vi "main_ctrl.vi"(8 "error in":errorcluster) -> (0 "error out":errorcluster caption="Error")   [LabVIEW 2013]
uses:
  <vilib>/Rock Robotics/WPI/DriverStation/WPI_DriverStationRobotMode2.ctl
  typedefs/Test/test data.ctl
  typedefs/Test/test controls.ctl
  typedefs/fg_typedef.ctl
  typedefs/Vision/vision enable.ctl
  typedefs/State Machine/subStates.ctl
  typedefs/State Machine/singleUseSubstate.ctl
  <vilib>/Rock Robotics/WPI/Solenoid/WPI_SolenoidValue.ctl
  <vilib>/Rock Robotics/WPI/Compressor/WPI_CompressorGetSetRefNum.vi
  <vilib>/Rock Robotics/WPI/RobotDrive/WPI_RobotDriveGetSetRefNum.vi
  <vilib>/Rock Robotics/WPI/RobotDrive/WPI_RobotDriveArcadeDrive_Standard(NoSaturation).vi
  <vilib>/Rock Robotics/WPI/Solenoid/WPI_SolenoidSetEnum.vi
  state machine master/Cancel State Machine - Pickup.vi
  state machine master/Cancel State Machine - Load.vi
  typedefs/Vision/vision data.ctl
panel:
  in  "Test\nControls":T1 {"Belts" scale=-1.0..1.0; "Arm" scale=-1.0..1.0; "Drive Train" scale=-1.0..1.0}
  out "Test Data":T2
  out "Robot Mode":T3
  out "Vision SPI":u32
  out "Vision IPS":dbl
  out "Main IPS":dbl
  out "Main SPI":u32
  # "Test Input/Output"
  # "MAIN CONTROL"
  # "holds robot control code - dual parallel state machine"
  # "SPI: milliseconds per iteration\nIPS: iterations per second"
  # "Pneumatics"
  # "Home Encoders"
  # "Manual Override"
  # "Joystick Control"
  # "Arm Safeties"
  # "Sensors"
  # "Drive Encoders"
  # "Pneumatics Commands"
  # "Arm Encoder"
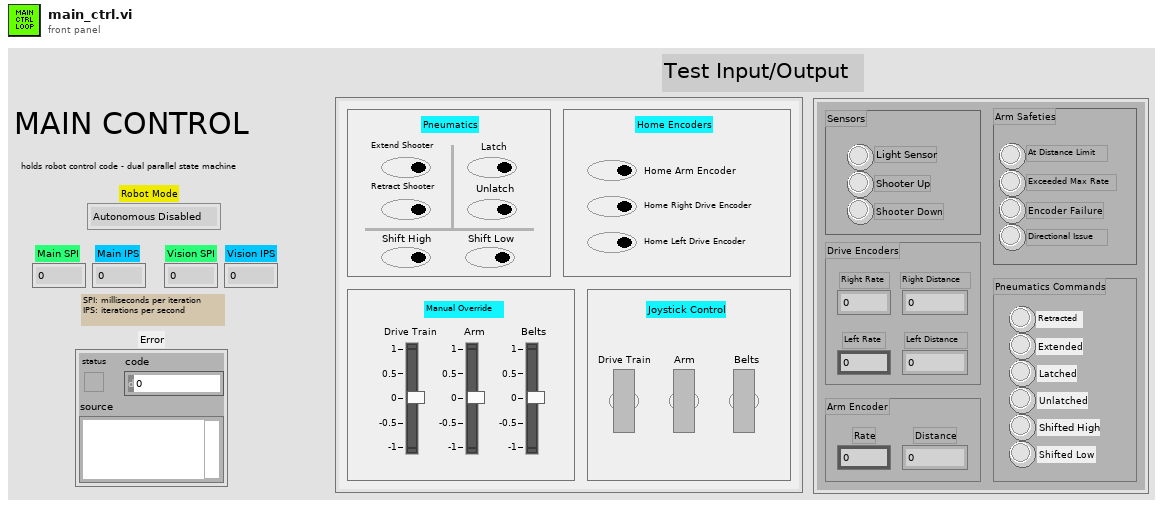
[diagram p1: front panel]
types:
  T1 = typedef "test controls.ctl" = cluster{"Drive Train":dbl, "Arm":dbl, "Belts":dbl, "Drive Train":bool, "Arm":bool, "Belts":bool, "Home Arm Encoder":bool, "Home Right Drive Encoder":bool, "Home Left Drive Encoder":bool, "Extend Shooter":bool, "Retract Shooter":bool, "Latch":bool, "Unlatch":bool, "Shift High":bool, "Shift Low":bool}
  T2 = typedef "test data.ctl" = cluster{"Light Sensor":bool, "Shooter Up":bool, "Shooter Down":bool, "Left Rate":dbl, "Left Distance":dbl, "Right Rate":dbl, "Right Distance":dbl, "Rate":dbl, "Distance":dbl, "At Distance Limit":bool, "Exceeded Max Rate":bool, "Encoder Failure":bool, "Directional Issue":bool, "Latched":bool, "Unlatched":bool, "Shifted High":bool, "Shifted Low":bool, "Extended":bool, "Retracted":bool}
  T3 = typedef "WPI_DriverStationRobotMode2.ctl" = enum16{"Autonomous Disabled", "Autonomous Enabled", "Teleop Disabled", "Teleop Enabled", "Timeout", "Finish", "Test Disabled", "Test Enabled"}
  T4 = typedef "fg_typedef.ctl" = enum16{"Get", "Set"}
  T5 = typedef "vision data.ctl" = cluster{"x":dbl, "y":dbl, "area":dbl, "width":dbl, "height":dbl, "Hot Goal Present?":bool, "distance":dbl}
  T6 = typedef "vision enable.ctl" = enum16{"Enable", "Disable", "Stop"}
  T7 = typedef "WPI_CameraDevRef.ctl" = cluster{"Camera Address":string, "CameraStatus":errorcluster, "Acquire Image Notifier":refnum<notifier>}
  T8 = typedef "IMAQ Image.ctl" = refnum<image>
  T9 = cluster{"Vision mSPI":u32, "Main mSPI":u32, "Dash mSPI":u32}
  T10 = typedef "WPI_RobotDriveDevRef.ctl" = cluster{"DevStatus":errorcluster, "Motors[]":T11[], "Square Inputs":bool, "Max Output":dbl, "Isochronous":bool}
  T11 = typedef "WPI_MotorControlDeviceRef.ctl" = cluster{"DeviceStatus":errorcluster, "Type":enum16{"PWM", "CAN"}, "PWM":cluster{"Digital Module":T12, "PWM Channel":T13, "DeadBand":T14}, "CAN":cluster{"Device Number":u8, "Control Mode":T15, "Semaphore":T16, "Max Vout":dbl}, "Invert":bool, "TransformRef":T17, "InvTransformRef":T17}
  T12 = typedef "FPGA_TypedefDigitalModule.ctl" = enum16{"Digital Module 1", "Digital Module 2"}
  T13 = typedef "FPGA_DIOPWMChannel.ctl" = enum8{"PWM 1", "PWM 2", "PWM 3", "PWM 4", "PWM 5", "PWM 6", "PWM 7", "PWM 8", "PWM 9", "PWM 10", "Invalid"}
  T14 = typedef "WPI_PWMDeadband.ctl" = cluster{"Name":string, "maxPositivePwm":i32, "minPositivePwm":i32, "centerPwm":i32, "maxNegativePwm":i32, "minNegativePwm":i32, "angularRange":u16}
  T15 = typedef "WPI_CANJaguar_ControlMode.ctl" = enum8{"Percent VBus", "Current", "Speed", "Position", "Voltage"}
  T16 = typedef "Semaphore RefNum" = refnum<k1>
  T17 = typedef "WPI_PWMTransform_ConPane.ctl" = refnum<vi>
  T18 = typedef "WPI_SolenoidDevRef.ctl" = cluster{"DevStatus":errorcluster, "Solenoid Module":T19, "Forward Solenoid Channel":T20, "Reverse Solenoid Channel":T20}
  T19 = typedef "FPGA_TypedefSolenoidModule.ctl" = enum16{"Solenoid Module 1", "Solenoid Module 2"}
  T20 = typedef "WPI_SolenoidChannel.ctl" = enum8{"Solenoid 1", "Solenoid 2", "Solenoid 3", "Solenoid 4", "Solenoid 5", "Solenoid 6", "Solenoid 7", "Solenoid 8", "Invalid"}
  T21 = typedef "WPI_CompressorDevRef.ctl" = cluster{"DevStatus":errorcluster, "DigitalInputDevRef":T22, "RelayDevRef":T24}
  T22 = typedef "WPI_DigitalInputDevRef.ctl" = cluster{"DevStatus":errorcluster, "DIO Channel":T23, "Digital Module":T12}
  T23 = typedef "FPGA_DIOChannel.ctl" = enum8{"DIO 1", "DIO 2", "DIO 3", "DIO 4", "DIO 5", "DIO 6", "DIO 7", "DIO 8", "DIO 9", "DIO 10", "DIO 11", "DIO 12", "DIO 13", "DIO 14", "Invalid"}
  T24 = typedef "WPI_RelayDevRef.ctl" = cluster{"DevStatus":errorcluster, "Relay Channel":T25, "Digital Module":T12, "Relay Direction":T26}
  T25 = typedef "FPGA_DIORelayChannel.ctl" = enum8{"Relay 1", "Relay 2", "Relay 3", "Relay 4", "Relay 5", "Relay 6", "Relay 7", "Relay 8", "Invalid"}
  T26 = typedef "WPI_RelayDirection.ctl" = enum16{"Both directions", "Forward only", "Reverse only"}
  T27 = typedef "WPI_SolenoidValue.ctl" = enum16{"Off", "On", "Forward", "Reverse"}
  T28 = typedef "singleUseSubstate.ctl" = enum16{"null", "wait", "shift high", "shift low", "extend shooter", "retract shooter", "latch", "unlatch", "end"}
  T29 = typedef "WPI_DriverStationDerivedRobotMode.ctl" = enum16{"Init", "Execute", "Stop"}
  T30 = typedef "subStates.ctl" = enum16{"null", "wait", "driver control", "auto", "manual override", "hold position", "rotate", "pickup", "pass", "load", "goto shoot", "shoot high goal", "shoot low goal", "cancel arm", "cancel shooter", "end", "test"}
  T31 = typedef "Loop 2 Datatype.ctl" = cluster{"State":T30, "Waiting Loop":i32, "State to Wait For":i32, "Loop ID":i32, "Exit Value":i32, "Joystick Y":dbl, "Joystick Z":dbl}
  T32 = typedef "Loop 1 Datatype.ctl" = cluster{"State":T30, "Waiting Loop":i32, "State to Wait For":i32, "Loop ID":i32, "Exit Value":i32}
  T33 = typedef "Loop 3 Datatype.ctl" = cluster{"State":T30, "Waiting Loop":i32, "State to Wait For":i32, "Loop ID":i32, "Exit Value":i32, "Joystick Y":dbl, "Tune Setpoint":cluster{"Increment":bool, "Decrement":bool}}
  T34 = typedef "Loop 0 Datatype.ctl" = cluster{"State":T30, "Waiting Loop":i32, "State to Wait For":i32, "Loop ID":i32, "Exit Value":i32, "X Axis":dbl, "Y Axis":dbl, "Z Axis":dbl}
  T35 = typedef "dashboard safety status data.ctl" = cluster{"At Distance Limit":bool, "Encoder Error":bool, "Excedded Rate Limit":bool, "Encoder Directional Issue":bool}
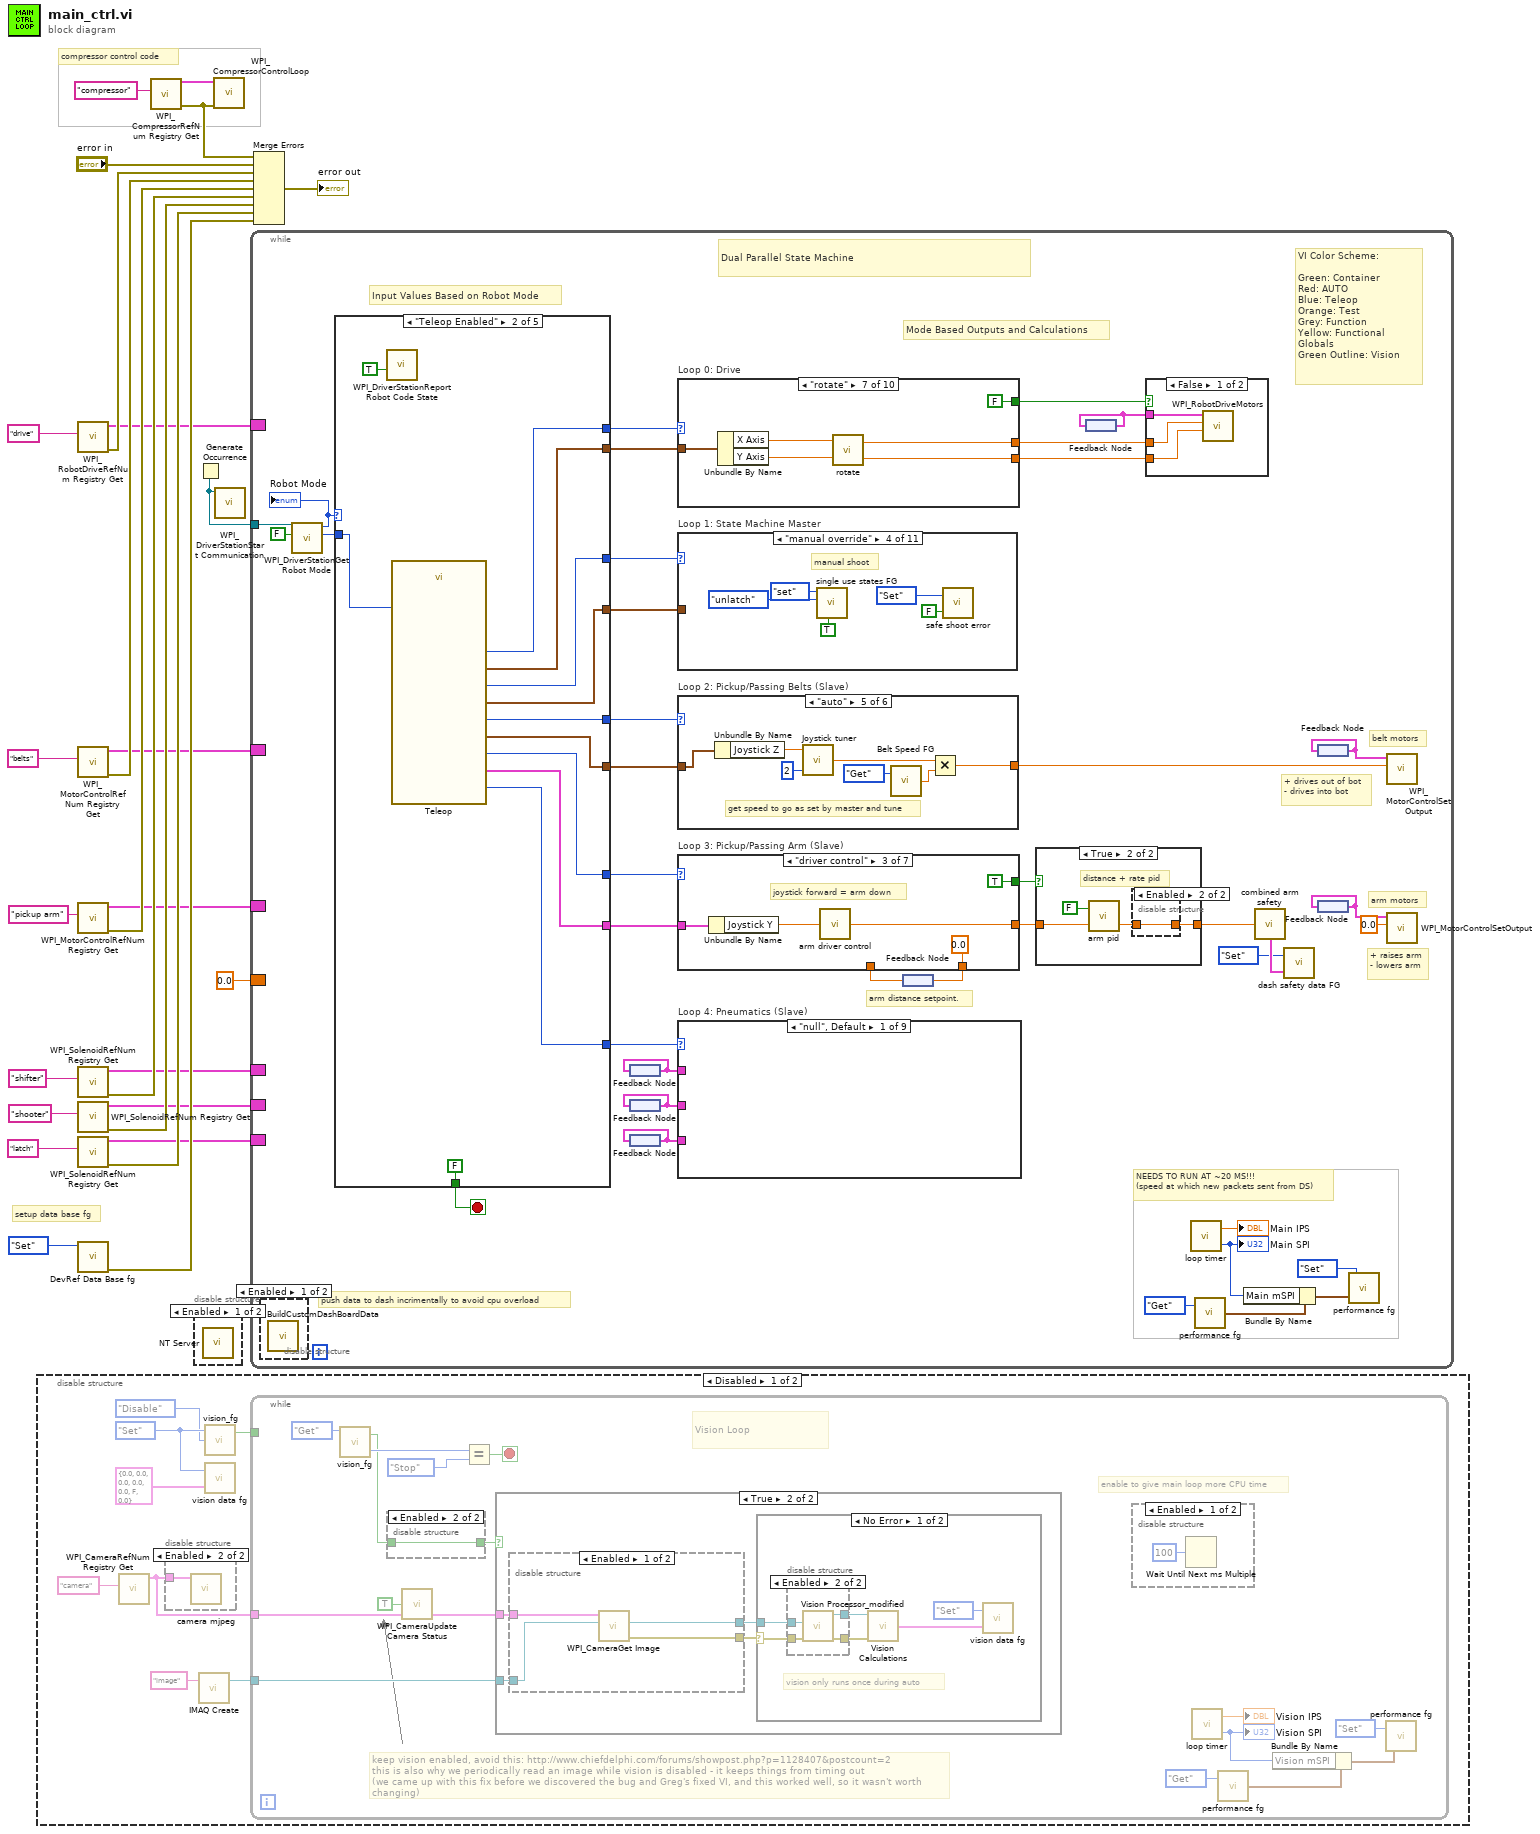
[diagram p0: block diagram]
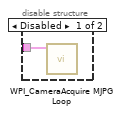
[diagram p3: hidden frame]
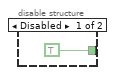
[diagram p4: hidden frame]
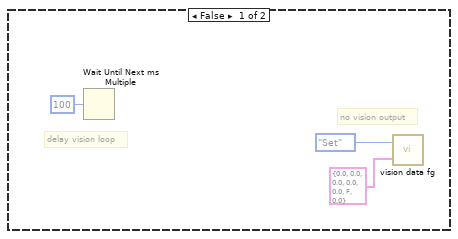
[diagram p6: hidden frame]
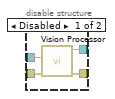
[diagram p7: hidden frame]
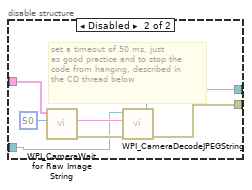
[diagram p9: hidden frame]
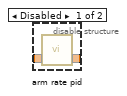
[diagram p12: hidden frame]
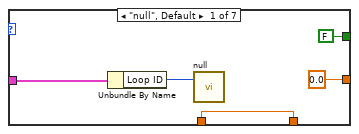
[diagram p13: hidden frame]
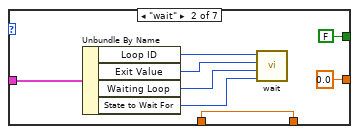
[diagram p14: hidden frame]
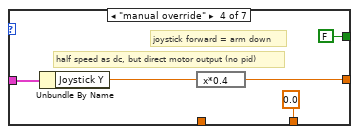
[diagram p15: hidden frame]
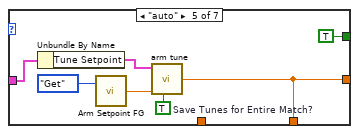
[diagram p16: hidden frame]
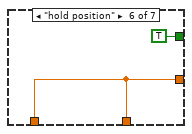
[diagram p17: hidden frame]
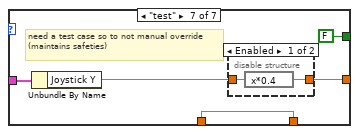
[diagram p18: hidden frame]
diagram:
  # "compressor control code"
  # "setup data base fg"
  n1 = disable-structure shown="Disabled" {
    frame Disabled {
      w33 = fg_typedef."Set" ("Enum")
      n2 = call <vilib>:"WPI_CameraRefNum Registry Get.vi"("refnum name"="camera") -> ("CameraDevRef"=w30:T7)  [unwired: 9 in, 1 out]
      n3 = disable-structure shown="Enabled" {
        disable-tunnel: w30 -> [w36 w37]
        frame Disabled {
          n4 = call <vilib>:"WPI_CameraAcquire MJPG Loop.vi"("CameraDevRef"=w36) -> ()  [unwired: 11 in]
        }
        frame Enabled {
          n5 = call "camera mjpeg.vi"("CameraDevRef"=w37) -> ()  [unwired: 11 in]
        }
      }
      n6 = call "IMAQ Create"("Image Name"="image") -> ("New Image"=w35:T8)  [unwired: 4 in, 1 out]
      n7 = call "vision_fg.vi"("Action"=vision_enable."Disable", "Menu"=w33) -> ("Enabled?"=w34:bool)  [unwired: 1 in, 1 out]
      n8 = call "vision data fg.vi"("Input"=T5 {"x"=0.0, "y"=0.0, "area"=0.0, "width"=0.0, "height"=0.0, "Hot Goal Present?"=FALSE, "distance"=0.0} ("Cluster"), "Menu"=w33) -> ()  [unwired: 1 out]
      n9 = while {
        tunnel: w35 -> [w52]
        tunnel: w30 -> [w51]
        tunnel: w34 -> [_]
        stop <- w53 stop-if-true
        # "keep vision enabled, avoid this: http://www.chiefdelphi.com/forums/showpost.php?p=1128407&postcount=2\nthis is also why we periodically read an image while vision is disabled - it keeps things from timing out\n(we came up with this fix before we discovered the bug and Greg's fixed VI, and this worked well, so it wasn't worth changing)"
        # "enable to give main loop more CPU time"
        # "Vision Loop"
        n10 = call "vision_fg.vi"("Menu"=fg_typedef."Get" ("Enum")) -> ("State Out"=w47:T6, "Enabled?"=w38:bool)  [unwired: 2 in]
        n11 = disable-structure shown="Enabled" {
          disable-tunnel: [TRUE w55] -> w39
          disable-tunnel: w38 -> [_ w55]
          frame Disabled {
          }
          frame Enabled {
          }
        }
        n12 = call <vilib>:"WPI_CameraUpdate Camera Status.vi"("CameraDevRef In"=w51, "Enable Vision"=TRUE) -> ("CameraDevRef Out"=w50:T7)  [unwired: 3 in]
        n13 = Equal?(x=w47, y=vision_enable."Stop") -> (x = y?=w53:bool)
        n14 = case shown="True" w39 {
          tunnel: w52 -> [_ w63]
          tunnel: w50 -> [_ w62]
          frame False {
            # "no vision output"
            # "delay vision loop"
            n15 = Wait Until Next ms Multiple(millisecond multiple=u32 100) -> ()  [unwired: 1 out]
            n16 = call "vision data fg.vi"("Input"=T5 {"x"=0.0, "y"=0.0, "area"=0.0, "width"=0.0, "height"=0.0, "Hot Goal Present?"=FALSE, "distance"=0.0} ("Cluster"), "Menu"=fg_typedef."Set" ("Enum")) -> ()  [unwired: 1 out]
          }
          frame True {
            n17 = disable-structure shown="Enabled" {
              disable-tunnel: w63 -> [w80 w84]
              disable-tunnel: w62 -> [w81 w86]
              disable-tunnel: [w79 w83] -> w61
              disable-tunnel: [w78 w82] -> w60
              frame Enabled {
                n18 = call <vilib>:"WPI_CameraGet Image.vi"("Image"=w80, "CameraDevRef"=w81) -> ("error out"=w78:errorcluster, "Image Out"=w79:T8)  [unwired: 7 in, 1 out]
              }
              frame Disabled {
                # "set a timeout of 50 ms, just\nas good practice and to stop the \ncode from hanging, described in \nthe CD thread below"
                n19 = call <vilib>:"WPI_CameraWait for Raw Image String.vi"("Timeout in ms (-1)"=50, "CameraDevRef"=w86) -> ("error out"=w88:errorcluster, "String"=w87:string)  [unwired: 3 in, 5 out]
                n20 = call <vilib>:"WPI_CameraDecodeJPEGString.vi"("error in"=w88, "Compressed Image"=w87, "Image In"=w84) -> ("error out"=w82:errorcluster, "Image Out"=w83:T8)  [unwired: 3 out]
              }
            }
            n21 = case shown="No Error" w60 {
              selector: w60 -> [w68 _]
              tunnel: w61 -> [w67 _]
              frame No Error {
                # "vision only runs once during auto"
                n22 = disable-structure shown="Enabled" {
                  disable-tunnel: w68 -> [w73 w76]
                  disable-tunnel: w67 -> [w72 w77]
                  disable-tunnel: [w71 w74] -> w66
                  disable-tunnel: [w70 w75] -> w65
                  frame Disabled {
                    n23 = call "Vision Processor.vi"("error in"=w73, "Image In"=w72) -> ("error out"=w70:errorcluster, "Image Out"=w71:T8)  [unwired: 5 in]
                  }
                  frame Enabled {
                    n24 = call "Vision Processor_modified.vi"("error in"=w76, "Image In"=w77) -> ("error out"=w75:errorcluster, "Image Out"=w74:T8)  [unwired: 5 in]
                  }
                }
                n25 = call "Vision Calculations.vi"("Image In"=w66, "error in"=w65) -> ("Vision Data"=w64:T5)  [unwired: 3 in]
                n26 = call "vision data fg.vi"("Input"=w64, "Menu"=fg_typedef."Set" ("Enum")) -> ()  [unwired: 1 out]
              }
              frame Error {
              }
            }
          }
        }
        n27 = disable-structure shown="Enabled" {
          frame Enabled {
            n28 = Wait Until Next ms Multiple(millisecond multiple=u32 100) -> ()  [unwired: 1 out]
          }
          frame Disabled {
          }
        }
        n29 = call "loop timer.vi"() -> ("IPS"=→"Vision IPS":dbl, "SPI"=w45:u32)  [unwired: 1 in]
        "Vision SPI" <- w45
        n30 = call "performance fg.vi"("Menu"=fg_typedef."Get") -> ("Output"=w43:T9)  [unwired: 1 in]
        n31 = Bundle By Name(cluster=w43, "Vision mSPI"=w45) -> (w42:T9)
        n32 = call "performance fg.vi"("Input"=w42, "Menu"=fg_typedef."Set") -> ()  [unwired: 1 out]
      }
    }
    frame Enabled {
      # "vision disabled"
    }
  }
  n33 = call <vilib>:"WPI_RobotDriveRefNum Registry Get.vi"("refnum name"="drive") -> ("error out"=w26:errorcluster, "RobotDriveDevRef"=w1:T10)  [unwired: 9 in]
  n34 = call <vilib>:"WPI_MotorControlRefNum Registry Get.vi"("refnum name"="belts") -> ("error out"=w25:errorcluster, "MotorControlDevRef"=w5:T11)  [unwired: 9 in]
  n35 = call <vilib>:"WPI_MotorControlRefNum Registry Get.vi"("refnum name"="pickup arm") -> ("error out"=w24:errorcluster, "MotorControlDevRef"=w9:T11)  [unwired: 9 in]
  n36 = call <vilib>:"WPI_SolenoidRefNum Registry Get.vi"("refnum name"="shifter") -> ("error out"=w23:errorcluster, "SolenoidDevRef"=w16:T18)  [unwired: 9 in]
  n37 = call <vilib>:"WPI_SolenoidRefNum Registry Get.vi"("refnum name"="shooter") -> ("error out"=w22:errorcluster, "SolenoidDevRef"=w3:T18)  [unwired: 9 in]
  n38 = call <vilib>:"WPI_SolenoidRefNum Registry Get.vi"("refnum name"="latch") -> ("error out"=w21:errorcluster, "SolenoidDevRef"=w4:T18)  [unwired: 9 in]
  n39 = call "DevRef Data Base fg.vi"("Menu"=fg_typedef."Set") -> ("error out"=w27:errorcluster)  [unwired: 3 in, 5 out]
  n40 = call <vilib>:"WPI_CompressorRefNum Registry Get.vi"("refnum name"="compressor") -> ("error out"=w8:errorcluster, "CompressorDevRef"=w17:T21)  [unwired: 9 in]
  n41 = disable-structure shown="Enabled" {
    frame Enabled {
      n42 = call <vilib>:"NT Server.vi"() -> ()  [unwired: 12 in]
    }
    frame Disabled {
    }
  }
  n43 = Generate Occurrence() -> (w14:refnum<k4>)
  n44 = call <vilib>:"WPI_CompressorControlLoop.vi"("error in (no error)"=w8, "CompressorDevRef"=w17) -> ()  [unwired: 10 in]
  n45 = call <vilib>:"WPI_DriverStationStart Communication.vi"("occurrence"=w14) -> ()  [unwired: 11 in]
  n46 = while {
    tunnel: w14 -> [w106]
    border: w1 -> [_]
    border: w16 -> [_]
    border: w4 -> [_]
    border: w3 -> [_]
    border: w5 -> [_]
    border: w9 -> [_]
    border: 0.0 ("setpoint") -> [_]
    stop <- w123 stop-if-true
    # "arm motors"
    # "arm distance setpoint."
    # "push data to dash incrimentally to avoid cpu overload"
    # "+ raises arm\n- lowers arm"
    # "+ drives out of bot\n- drives into bot"
    # "belt motors"
    # "VI Color Scheme:\n\nGreen: Container\nRed: AUTO\nBlue: Teleop\nOrange: Test \nGrey: Function\nYellow: Functional Globals\nGreen Outline: Vision"
    # "Input Values Based on Robot Mode"
    # "Mode Based Outputs and Calculations"
    # "NEEDS TO RUN AT ~20 MS!!!\n(speed at which new packets sent from DS)"
    # "Dual Parallel State Machine"
    n47 = disable-structure shown="Enabled" {
      frame Enabled {
        n48 = call "BuildCustomDashBoardData.vi"() -> ()  [unwired: 12 in]
      }
      frame Disabled {
      }
    }
    n49 = call <vilib>:"WPI_DriverStationGet Robot Mode.vi"("Finish"=FALSE, "DS Occurrence"=w106) -> ("Call Context"=w105:T29, "Robot Mode"=w104:T3)  [unwired: 8 out]
    "Robot Mode" <- w104
    n50 = case shown="\"Teleop Enabled\"" w104 {
      tunnel: [w305 w320 w329 w337 w343] -> w108
      tunnel: w105 -> [w298 w316 w332 _ _]
      tunnel: [w303 w319 w331 w337 w343] -> w125
      tunnel: [w299 w317 w323 singleUseSubstate."null" ("SubState 5") singleUseSubstate."end" ("SubState 5")] -> w124
      tunnel: [FALSE FALSE FALSE FALSE TRUE] -> w123
      tunnel: [w307 w315 w327 w337 w343] -> w94
      tunnel: [w306 w314 w328 _ _] -> w117
      tunnel: [w304 w313 w330 _ _] -> w116
      tunnel: [w302 w312 w326 _ _] -> w115
      tunnel: [w300 w311 w324 _ _] -> w113
      tunnel: [w301 w310 w325 w337 w343] -> w93
      frame "Autonomous Enabled" {
        n51 = call <vilib>:"WPI_DriverStationReport Robot Code State.vi"("Autonomous"=TRUE) -> ()  [unwired: 10 in, 1 out]
        n52 = call "Autonomous.vi"("Call Context"=w298) -> ("SubState 2"=w303:T30, "Loop 2 Data"=w302:T31, "SubState 1"=w305:T30, "Loop 1 Data"=w304:T32, "Loop 3 Data"=w300:T33, "SubState 0"=w307:T30, "SubState 3"=w301:T30, "Loop 0 Data"=w306:T34, "SubState 4"=w299:T28)  [unwired: 2 in]
      }
      frame "Teleop Enabled" {
        n53 = call <vilib>:"WPI_DriverStationReport Robot Code State.vi"("TeleOp"=TRUE) -> ()  [unwired: 10 in, 1 out]
        n54 = call "Teleop.vi"("Call Context"=w316) -> ("SubState 3"=w310:T30, "SubState 4"=w317:T28, "Loop 3 Data"=w311:T33, "SubState 0"=w315:T30, "Loop 1 Data"=w313:T32, "Loop 0 Data"=w314:T34, "SubState 1"=w320:T30, "Loop 2 Data"=w312:T31, "SubState 2"=w319:T30)  [unwired: 10 in]
      }
      frame "Test Enabled" {
        n55 = call <vilib>:"WPI_DriverStationReport Robot Code State.vi"("Test"=TRUE) -> ()  [unwired: 10 in, 1 out]
        n56 = call "Test.vi"("Test Controls"="Test\nControls", "Call Context"=w332) -> ("Loop 2 Data"=w326:T31, "SubState 2"=w331:T30, "Loop 1 Data"=w330:T32, "SubState 1"=w329:T30, "SubState 3"=w325:T30, "Loop 0 Data"=w328:T34, "Loop 3 Data"=w324:T33, "SubState 0"=w327:T30, "SubState 4"=w323:T28, "Test Data"=→"Test Data":T2)
      }
      frame "Autonomous Disabled", "Teleop Disabled", "Timeout", "Test Disabled" {
        w337 = subStates."null" ("SubState 0")
        # "set all loops to null"
        # "make sure to disable vision\nwe don't need it here"
        # "robot disabled, timeout"
        n57 = call <vilib>:"WPI_DriverStationReport Robot Code State.vi"("Disabled"=TRUE) -> ()  [unwired: 10 in, 1 out]
        n58 = call "vision_fg.vi"("Action"=vision_enable."Disable", "Menu"=fg_typedef."Set") -> ()  [unwired: 1 in, 2 out]
      }
      frame "Finish" {
        w343 = subStates."end" ("Loop State")
        # "Stop All Loops"
        # "stop the while loop"
        # "stop DS comms"
        # "stop vision loop"
        n59 = call <vilib>:"WPI_DriverStationStop Communication.vi"("StopCommunication"=TRUE) -> ()  [unwired: 10 in, 1 out]
        n60 = call "vision_fg.vi"("Action"=vision_enable."Stop", "Menu"=fg_typedef."Set") -> ()  [unwired: 1 in, 2 out]
      }
    }
    n61 = feedback #1() -> (w114:T18)
    n62 = feedback-in #1(w114) -> ()
    n63 = feedback #2() -> (w100:T18)
    n64 = feedback-in #2(w100) -> ()
    n65 = feedback #3() -> (w99:T18)
    n66 = feedback-in #3(w99) -> ()
    n67 = case "Loop 0: Drive" shown="\"rotate\"" w94 {
      tunnel: w117 -> [w184 w187 w197 w209 w217 w220 w226 _ w239 _]
      tunnel: [w183 w186 w196 w206 w214 w222 w228 w230 0.0 ("X Axis") w241] -> w111
      tunnel: [w183 w186 w195 w205 w213 w221 w227 w229 w238 w241] -> w110
      tunnel: [FALSE FALSE TRUE FALSE FALSE FALSE FALSE FALSE TRUE FALSE] -> w112
      frame "null", Default {
        w183 = 0.0 ("X Axis")
        n68 = Unbundle By Name(w184) -> ("Loop ID"=w182:i32)
        n69 = call "null.vi"("This Loop ID"=w182) -> ()  [unwired: 2 in]
      }
      frame "wait" {
        w186 = 0.0 ("X Axis")
        n70 = Unbundle By Name(w187) -> ("Loop ID"=w191:i32, "Exit Value"=w190:i32, "Waiting Loop"=w189:i32, "State to Wait For"=w188:i32)
        n71 = call "wait.vi"("State to wait for"=w188, "Waiting Loop ID"=w189, "time (ms)"=w190, "Current Loop ID"=w191) -> ()  [unwired: 1 out]
      }
      frame "driver control" {
        n72 = Unbundle By Name(w197) -> ("X Axis"=w193:dbl, "Y Axis"=w194:dbl)
        n73 = disable-structure shown="Enabled" {
          disable-tunnel: w193 -> [w201 w203]
          disable-tunnel: w194 -> [w200 w202]
          disable-tunnel: [w199 w203] -> w196
          disable-tunnel: [w198 w202] -> w195
          frame Disabled {
            n74 = call "calc arcade drive pwm.vi"("Y axis value"=w200, "X axis value"=w201) -> ("Right Speed"=w198:dbl, "Left Speed"=w199:dbl)  [unwired: 1 in, 1 out]
          }
          frame Enabled {
          }
        }
      }
      frame "manual override" {
        n75 = Unbundle By Name(w209) -> ("X Axis"=w208:dbl, "Y Axis"=w207:dbl)
        n76 = expression code="x/2"(w208) -> (w206:dbl)
        n77 = expression code="x/2"(w207) -> (w205:dbl)
      }
      frame "hold position" {
        n78 = Unbundle By Name(w217) -> ("X Axis"=w216:dbl, "Y Axis"=w215:dbl)
        n79 = call "closed drive.vi"("Acrade Drive?"=TRUE, "Y axis value (Left)"=w215, "X axis value (Right)"=w216, "Threshold (.4)"=0.4) -> ("right"=w213:dbl, "left"=w214:dbl)
      }
      frame "auto" {
        n80 = Unbundle By Name(w220) -> ("X Axis"=w218:dbl)
        n81 = call "autoDrive.vi"("Distance"=w218) -> ("right speed"=w221:dbl, "left speed"=w222:dbl)  [unwired: 2 in, 1 out]
      }
      frame "rotate" {
        n82 = Unbundle By Name(w226) -> ("X Axis"=w225:dbl, "Y Axis"=w224:dbl)
        n83 = call "rotate.vi"("Rate"=w224, "Angle"=w225) -> ("right speed"=w227:dbl, "left speed"=w228:dbl)  [unwired: 1 in, 1 out]
      }
      frame "goto shoot" {
        n84 = disable-structure shown="Enabled" {
          disable-tunnel: [w233 _] -> w230
          disable-tunnel: [w232 _] -> w229
          frame Disabled {
            # "consider implimenting closed hold with drive"
            n85 = call "vision data fg.vi"("Menu"=fg_typedef."Get") -> ("Output"=w234:T5)  [unwired: 1 in]
            n86 = call "goto location.vi"("Image Data"=w234) -> ("left speed"=w233:dbl, "right speed"=w232:dbl)
          }
          frame Enabled {
            # "not going to do this"
          }
        }
      }
      frame "test" {
        n87 = Unbundle By Name(w239) -> ("Y Axis"=w238:dbl)
      }
      frame "end" {
        w241 = 0.0 ("X Axis")
      }
    }
    n88 = case "Loop 1: State Machine Master" shown="\"manual override\"" w108 {
      tunnel: w116 -> [w284 w285 _ _ _ _ _ _ _ _ _]
      frame "null", Default {
        n89 = Unbundle By Name(w284) -> ("Loop ID"=w283:i32)
        n90 = call "null.vi"("This Loop ID"=w283) -> ()  [unwired: 2 in]
      }
      frame "wait" {
        n91 = Unbundle By Name(w285) -> ("Loop ID"=w289:i32, "Exit Value"=w288:i32, "Waiting Loop"=w287:i32, "State to Wait For"=w286:i32)
        n92 = call "wait.vi"("State to wait for"=w286, "Waiting Loop ID"=w287, "time (ms)"=w288, "Current Loop ID"=w289) -> ()  [unwired: 1 out]
      }
      frame "auto" {
        # "A State Machine for Auto"
        n93 = call "Auto State Machine.vi"() -> ()  [unwired: 12 in]
      }
      frame "manual override" {
        # "manual shoot"
        n94 = call "single use states FG.vi"("exit in"=TRUE, "substate"=singleUseSubstate."unlatch", "menu (get)"=enum16{"set", "get"}."set") -> ()  [unwired: 5 in, 4 out]
        n95 = call "safe shoot error.vi"("Can Shoot Safely?"=FALSE, "Menu"=fg_typedef."Set") -> ()  [unwired: 1 out]
      }
      frame "pickup" {
        # "A State Machine for Pickup"
        n96 = call "Pickup State Machine.vi"() -> ()  [unwired: 12 in]
      }
      frame "pass" {
        # "A State Machine for Passing"
        n97 = call "Pass State Machine.vi"() -> ()  [unwired: 12 in]
      }
      frame "load" {
        # "ball can now (after this) be high or low goal shot"
        # "A State Machine for Loading"
        n98 = call "Load State Machine.vi"() -> ()  [unwired: 12 in]
      }
      frame "shoot high goal" {
        # "A State Machine for High Goal Shooting"
        n99 = call "Shoot High Goal State Machine.vi"() -> ()  [unwired: 12 in]
      }
      frame "shoot low goal" {
        # "A State Machine for Low Goal Shooting"
        n100 = call "Shoot Low Goal State Machine.vi"() -> ()  [unwired: 12 in]
      }
      frame "cancel arm" {
        # "A State Machine for Canceling Pickup"
        n101 = disable-structure shown="Disabled" {
          frame Disabled {
            n102 = call "Cancel State Machine.vi"("What to Cancel"=enum16{"Pickup", "Load"}."Pickup") -> ()
          }
          frame Enabled {
          }
        }
        n103 = call-poly "Cancel State Machine - Polymorphic.vi"() -> ()  [unwired: 1 in]
      }
      frame "cancel shooter" {
        # "A State Machine for Canceling Loading"
        n104 = disable-structure shown="Disabled" {
          frame Disabled {
            n105 = call "Cancel State Machine.vi"("What to Cancel"=enum16{"Pickup", "Load"}."Load") -> ()
          }
          frame Enabled {
          }
        }
        n106 = call-poly "Cancel State Machine - Polymorphic.vi"() -> ()  [unwired: 1 in]
      }
    }
    n107 = case "Loop 2: Pickup/Passing Belts (Slave)" shown="\"auto\"" w125 {
      tunnel: w115 -> [w259 w263 w270 w273 w280 w282]
      tunnel: [0.0 ("output") 0.0 ("output") w268 w271 w277 w281] -> w101
      frame "null", Default {
        # "must stay disabled, it caused errors"
        n108 = disable-structure shown="Disabled" {
          disable-tunnel: w259 -> [w261 _]
          frame Disabled {
            n109 = Unbundle By Name(w261) -> ("Loop ID"=w260:i32)
            n110 = call "null.vi"("This Loop ID"=w260) -> ()  [unwired: 2 in]
          }
          frame Enabled {
          }
        }
      }
      frame "wait" {
        n111 = Unbundle By Name(w263) -> ("Loop ID"=w267:i32, "Exit Value"=w266:i32, "Waiting Loop"=w265:i32, "State to Wait For"=w264:i32)
        n112 = call "wait.vi"("State to wait for"=w264, "Waiting Loop ID"=w265, "time (ms)"=w266, "Current Loop ID"=w267) -> ()  [unwired: 1 out]
      }
      frame "driver control" {
        # "which joystick? should be specified in name."
        # "joystick forward = out of bot"
        n113 = Unbundle By Name(w270) -> ("Joystick Y"=w269:dbl)
        n114 = Negate(x=w269) -> (-x=w268:dbl)
      }
      frame "manual override" {
        # "essentially driver control, but 1/2 speed?"
        # "joystick forward = out of bot"
        n115 = Unbundle By Name(w273) -> ("Joystick Y"=w272:dbl)
        n116 = expression code="-x/2"(w272) -> (w271:dbl)
      }
      frame "auto" {
        # "get speed to go as set by master and tune"
        n117 = Unbundle By Name(w280) -> ("Joystick Z"=w278:dbl)
        n118 = call "Joystick tuner.vi"("Joystick Z"=w278, "Loop ID"=2) -> ("Output"=w276:dbl)  [unwired: 7 in]
        n119 = call "Belt Speed FG.vi"("Menu"=fg_typedef."Get") -> ("Speed Out"=w275:dbl)  [unwired: 1 in]
        n120 = Multiply(x=w276, y=w275) -> (x*y=w277:dbl)
      }
      frame "test" {
        n121 = Unbundle By Name(w282) -> ("Joystick Y"=w281:dbl)
      }
    }
    n122 = case "Loop 4: Pneumatics (Slave)" shown="\"null\", Default" w124 {
      tunnel: w114 -> [_ _ w243 w244 _ _ _ _ _]
      tunnel: w100 -> [_ _ _ _ w246 w248 _ _ w256]
      tunnel: w99 -> [_ _ _ _ _ _ w250 w252 w254]
      frame "null", Default {
      }
      frame "wait" {
      }
      frame "shift high" {
        n123 = call-poly <vilib>:"WPI_SolenoidSet.vi"("Value"=WPI_SolenoidValue."Forward", "SolenoidDevRef"=w243) -> ()  [unwired: 8 in, 2 out]
      }
      frame "shift low" {
        n124 = call-poly <vilib>:"WPI_SolenoidSet.vi"("Value"=WPI_SolenoidValue."Reverse", "SolenoidDevRef"=w244) -> ()  [unwired: 8 in, 2 out]
      }
      frame "extend shooter" {
        n125 = call-poly <vilib>:"WPI_SolenoidSet.vi"("Value"=WPI_SolenoidValue."Forward", "SolenoidDevRef"=w246) -> ()  [unwired: 8 in, 2 out]
      }
      frame "retract shooter" {
        n126 = call-poly <vilib>:"WPI_SolenoidSet.vi"("Value"=WPI_SolenoidValue."Reverse", "SolenoidDevRef"=w248) -> ()  [unwired: 8 in, 2 out]
      }
      frame "latch" {
        # "When the latch piston\nis reversed, the latch\nis closed. When the\nlatch piston is\nextended, the latch is\nopen."
        n127 = call-poly <vilib>:"WPI_SolenoidSet.vi"("Value"=WPI_SolenoidValue."Reverse", "SolenoidDevRef"=w250) -> ()  [unwired: 8 in, 2 out]
      }
      frame "unlatch" {
        # "When the latch piston\nis reversed, the latch\nis closed. When the\nlatch piston is\nextended, the latch is\nopen."
        n128 = call-poly <vilib>:"WPI_SolenoidSet.vi"("Value"=WPI_SolenoidValue."Forward", "SolenoidDevRef"=w252) -> ()  [unwired: 8 in, 2 out]
      }
      frame "end" {
        # "retract shooter and unlatch"
        n129 = call-poly <vilib>:"WPI_SolenoidSet.vi"("Value"=WPI_SolenoidValue."Reverse", "SolenoidDevRef"=w256) -> ()  [unwired: 8 in, 2 out]
        n130 = call-poly <vilib>:"WPI_SolenoidSet.vi"("Value"=WPI_SolenoidValue."Forward", "SolenoidDevRef"=w254) -> ()  [unwired: 8 in, 2 out]
      }
    }
    n131 = feedback #4() -> (w95:dbl)
    n132 = case "Loop 3: Pickup/Passing Arm (Slave)" shown="\"driver control\"" w93 {
      tunnel: w113 -> [w139 w143 w151 w157 w164 _ w171]
      tunnel: [FALSE FALSE TRUE FALSE TRUE TRUE FALSE] -> w98
      tunnel: [0.0 ("output") 0.0 ("output") w150 w155 w158 w165 w167] -> w97
      tunnel: [w136 w140 0.0 ("setpoint") 0.0 ("setpoint") w158 w165 w168] -> w96
      tunnel: w95 -> [w136 w140 _ _ _ w165 w168]
      frame "null", Default {
        n133 = Unbundle By Name(w139) -> ("Loop ID"=w135:i32)
        n134 = call "null.vi"("This Loop ID"=w135) -> ()  [unwired: 2 in]
      }
      frame "wait" {
        n135 = Unbundle By Name(w143) -> ("Loop ID"=w147:i32, "Exit Value"=w146:i32, "Waiting Loop"=w145:i32, "State to Wait For"=w144:i32)
        n136 = call "wait.vi"("State to wait for"=w144, "Waiting Loop ID"=w145, "time (ms)"=w146, "Current Loop ID"=w147) -> ()  [unwired: 1 out]
      }
      frame "driver control" {
        # "joystick forward = arm down"
        n137 = Unbundle By Name(w151) -> ("Joystick Y"=w149:dbl)
        n138 = call "arm driver control.vi"("Joystick Y"=w149) -> ("Setpoint"=w150:dbl)
      }
      frame "manual override" {
        # "half speed as dc, but direct motor output (no pid)"
        # "joystick forward = arm down"
        n139 = Unbundle By Name(w157) -> ("Joystick Y"=w156:dbl)
        n140 = expression code="x*0.4"(w156) -> (w155:dbl)
      }
      frame "auto" {
        w159 = TRUE  # Save Tunes for Entire Match?
        n141 = Unbundle By Name(w164) -> ("Tune Setpoint"=w161:cluster{"Increment":bool, "Decrement":bool})
        n142 = call "Arm Setpoint FG.vi"("Menu"=fg_typedef."Get") -> ("Setpoint Out"=w160:dbl)  [unwired: 1 in]
        n143 = call "arm tune.vi"("Tune Data"=w161, "Setpoint"=w160, "Save Tunes for Entire Match?"=w159) -> ("Tuned Setpoint"=w158:dbl)  [unwired: 4 in]
      }
      frame "hold position" {
      }
      frame "test" {
        # "need a test case so to not manual override\n(maintains safeties)"
        n144 = Unbundle By Name(w171) -> ("Joystick Y"=w170:dbl)
        n145 = disable-structure shown="Enabled" {
          disable-tunnel: w170 -> [w173 w174]
          disable-tunnel: [w172 w174] -> w167
          frame Enabled {
            n146 = expression code="x*0.4"(w173) -> (w172:dbl)
          }
          frame Disabled {
          }
        }
      }
    }
    n147 = feedback-in #4(w96) -> ()
    n148 = case shown="True" w98 {
      tunnel: w97 -> [w127 w130]
      tunnel: [w127 w128] -> w90
      frame False {
        # "open loop"
      }
      frame True {
        # "distance + rate pid"
        n149 = call "arm pid.vi"("Setpoint"=w130, "Autotune?"=FALSE) -> ("Output"=w129:dbl)  [unwired: 1 in]
        n150 = disable-structure shown="Enabled" {
          disable-tunnel: w129 -> [w133 w134]
          disable-tunnel: [w132 w134] -> w128
          frame Disabled {
            n151 = call "arm rate pid.vi"("Rate In"=w133) -> ("Rate Out"=w132:dbl)  [unwired: 2 in]
          }
          frame Enabled {
          }
        }
      }
    }
    n152 = feedback #5() -> (w109:T10)
    n153 = feedback-in #5(w109) -> ()
    n154 = case shown="False" w112 {
      tunnel: w111 -> [w176 w180]
      tunnel: w110 -> [w175 w179]
      tunnel: w109 -> [w177 w178]
      frame False {
        n155 = call <vilib>:"WPI_RobotDriveMotors.vi"("RightSpeed"=w175, "LeftSpeed"=w176, "RobotDriveDevRef"=w177) -> ()  [unwired: 6 in, 3 out]
      }
      frame True {
        n156 = call-poly <vilib>:"WPI_RobotDriveArcadeDrive.vi"("Y axis value"=w179, "X axis value"=w180, "RobotDriveDevRef"=w178) -> ()  [unwired: 6 in, 3 out]
      }
    }
    n157 = call "loop timer.vi"() -> ("IPS"=→"Main IPS":dbl, "SPI"=w122:u32)  [unwired: 1 in]
    "Main SPI" <- w122
    n158 = call "performance fg.vi"("Menu"=fg_typedef."Get") -> ("Output"=w119:T9)  [unwired: 1 in]
    n159 = Bundle By Name(cluster=w119, "Main mSPI"=w122) -> (w118:T9)
    n160 = call "combined arm safety.vi"("Input"=w90) -> ("Safety Data"=w92:T35)  [unwired: 13 in, 1 out]
    n161 = call "dash safety data FG.vi"("Safety Data"=w92, "Menu"=fg_typedef."Set") -> ()  [unwired: 1 out]
    n162 = feedback #6() -> (w103:T11)
    n163 = feedback-in #6(w103) -> ()
    n164 = feedback #7() -> (w102:T11)
    n165 = feedback-in #7(w102) -> ()
    n166 = call "performance fg.vi"("Input"=w118, "Menu"=fg_typedef."Set") -> ()  [unwired: 1 out]
    n167 = call <vilib>:"WPI_MotorControlSetOutput.vi"("Output"=w101, "MotorControlDevRef"=w103) -> ()  [unwired: 7 in, 3 out]
    n168 = call <vilib>:"WPI_MotorControlSetOutput.vi"("Output"=0.0, "MotorControlDevRef"=w102) -> ()  [unwired: 7 in, 3 out]
  }
  n169 = Merge Errors(w8, "error in", w26, w25, w24, w23, w22, w21, w27) -> (→"error out":errorcluster)
